vi "UNITTEST-JSON-RPC-speed.vi"() -> ()   [LabVIEW 2019]
uses:
  04e4e71a-2c9d-4a45-8856-8c47119f5aac.vi
  ade66e49-40a9-47ce-a3dc-a089706bbdf8.vi
  a436de84-ac6b-4cd3-aef1-f9052b7ecc75.vi
  <vilib>/JDP Science/JSONtext/Make JSON Array.vi
  ade66e49-40a9-47ce-a3dc-a089706bbdf8.vi/90f3c966-384a-435e-906f-d07b11c8ef14.vi
  ade66e49-40a9-47ce-a3dc-a089706bbdf8.vi/38582f25-58de-4f8a-9f84-1f7c2dd61a81.vi
  a436de84-ac6b-4cd3-aef1-f9052b7ecc75.vi/cb0652dd-417e-4c76-946e-40e384de6030.vi
  <vilib>/JDP Science/JSONtext/Variant to JSON Text.vi
  <vilib>/JDP Science/JSONtext/support/Format JSON Array Text.vi
  <vilib>/Utility/Data Type/Get Type Information.vi
  <vilib>/JDP Science/JSONtext/JSON text to Variant.vi
  <vilib>/JDP Science/JSONtext/LVClass Serializer/JSONtext LVClass Serializer.lvclass
  JSON-RPC/JSON-RPC.lvlib
panel:
  out "Data in":dbl[](array[numeric])
  out "error out":errorcluster
  out "Data out":dbl[](array[numeric])
  in  "flatten":bool
  out "flatten":dbl
  out "unflatten":dbl
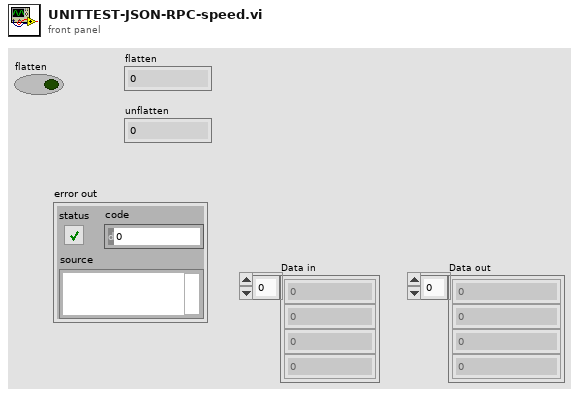
[diagram p1: front panel]
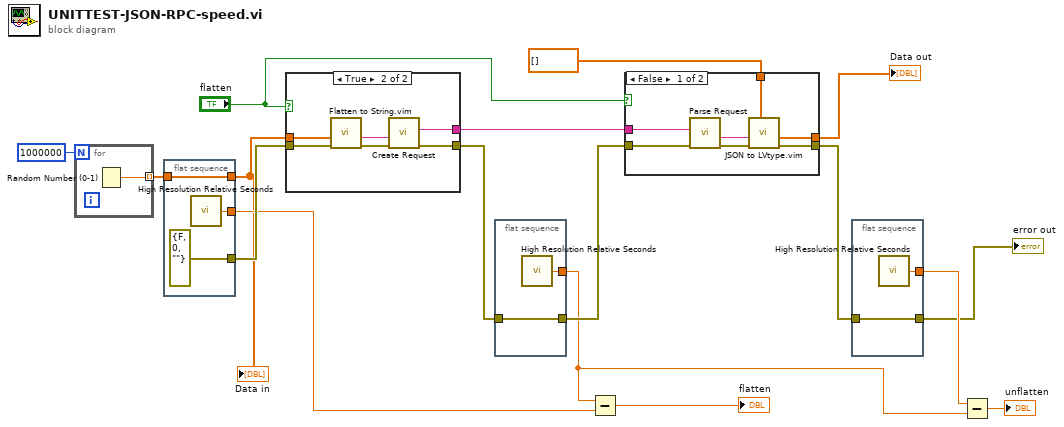
[diagram p0: block diagram]
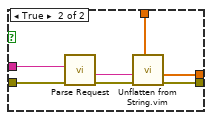
[diagram p2: hidden frame]
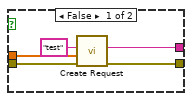
[diagram p3: hidden frame]
diagram:
  n1 = for {
    N: 1000000 -> [_]
    tunnel: [w18] -> w13 mode=indexing
    n2 = Random Number (0-1)() -> (number: 0 to 1=w18:dbl)
  }
  n3 = flat-sequence {
    tunnel: w13 -> [w21]
    tunnel: [w21] -> w3
    tunnel: [errorcluster {"status"=FALSE, "code"=0, "source"=""} ("error in (no error)")] -> w17
    tunnel: [w19] -> w12
    frame #0 {
      n4 = call <vilib>:"High Resolution Relative Seconds.vi"() -> ("relative seconds"=w19:dbl)
    }
  }
  n5 = case shown="True" "flatten" {
    tunnel: w3 -> [w22 w32]
    tunnel: w17 -> [w26 w31]
    tunnel: [w24 w28] -> w16
    tunnel: [w25 w29] -> w2
    frame False {
      n6 = call "Create Request.vi"("error in (no error)"=w26, "params"=w22, "method"="test") -> ("error out"=w24:errorcluster, "<JSON> Requests"=w25:string)  [unwired: 6 in, 1 out]
    }
    frame True {
      n7 = call "Flatten to String.vim"("error in (no error)"=w31, "Data in"=w32) -> ("error out"=w30:errorcluster, "<JSON>"=w27:string)  [unwired: 8 in]
      n8 = call "Create Request.vi"("error in (no error)"=w30, "params"=w27) -> ("error out"=w28:errorcluster, "<JSON> Requests"=w29:string)  [unwired: 7 in, 1 out]
    }
  }
  n9 = flat-sequence {
    tunnel: [w34] -> w15
    tunnel: w16 -> [w34]
    tunnel: [w33] -> w10
    frame #0 {
      n10 = call <vilib>:"High Resolution Relative Seconds.vi"() -> ("relative seconds"=w33:dbl)
    }
  }
  n11 = Subtract(x=w10, y=w12) -> (x-y=→"flatten":dbl)
  n12 = case shown="False" "flatten" {
    tunnel: w15 -> [w41 w45]
    tunnel: [w36 w48] -> w14
    tunnel: w2 -> [w40 w46]
    tunnel: dbl[] [] -> [w39 w42]
    tunnel: [w35 w47] -> w1
    frame False {
      n13 = call "Parse Request.vi"("error in (no error)"=w41, "<JSON> Requests"=w40) -> ("error out"=w37:errorcluster, "Params"=w38:string)  [unwired: 6 in, 2 out]
      n14 = call "JSON to LVtype.vim"("type"=w39, "error in (no error)"=w37, "JSON Data in"=w38) -> ("error out"=w36:errorcluster, "Data out"=w35:dbl[])  [unwired: 7 in]
    }
    frame True {
      n15 = call "Parse Request.vi"("error in (no error)"=w45, "<JSON> Requests"=w46) -> ("error out"=w43:errorcluster, "Params"=w44:string)  [unwired: 6 in, 2 out]
      n16 = call "Unflatten from String.vim"("type"=w42, "error in (no error)"=w43, "<JSON>"=w44) -> ("error out"=w48:errorcluster, "Data out"=w47:dbl[])  [unwired: 7 in]
    }
  }
  "Data out" <- w1
  n17 = flat-sequence {
    tunnel: [w50] -> w6
    tunnel: w14 -> [w50]
    tunnel: [w49] -> w11
    frame #0 {
      n18 = call <vilib>:"High Resolution Relative Seconds.vi"() -> ("relative seconds"=w49:dbl)
    }
  }
  n19 = Subtract(x=w11, y=w10) -> (x-y=→"unflatten":dbl)
  "error out" <- w6
  "Data in" <- w3
